vi "EnumControls.vi"(7 "Seasons":enum8{"Spring", "Summer", "Fall", "Winter"}(ring), 10 "Months":T1(ring)=enum."December", 11 "Colors":enum16{"Red", "Green", "Blue"}(ring)=enum."Green") -> ()   [LabVIEW 2012]
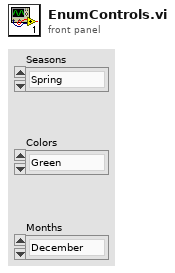
[diagram p1: front panel]
types:
  T1 = enum32{"<Invalid>", "January", "February", "March", "April", "May", "June", "July", "August", "September", "October", "November", "December"}
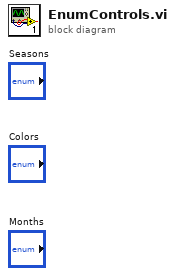
[diagram p0: block diagram]
diagram:
